vi "Autonomous Independent.vi"() -> ()   [LabVIEW 2019]
doc: "This VI is called when autonomous begins, and will automatically be terminated when autonomous ends. You can carry out timed or sensor driven robot movement independently without needing to return to the caller."
uses:
  <vilib>/Rock Robotics/WPI/Utilities/WPI_GetSetVariantRefNum.vi
  <vilib>/Rock Robotics/Network Tables/NT Read String.vi
  <vilib>/Rock Robotics/Network Tables/NT Write Numeric Array.vi
  Robot Global Data.vi
  <vilib>/Rock Robotics/WPI/RobotDrive/WPI_RobotDriveArcadeDrive_Standard(NoSaturation).vi
panel:
  out "time":u32
  # "Be sure to right-click and choose Data Operations>>Make Current Value default if you want to save the array values with the VI"
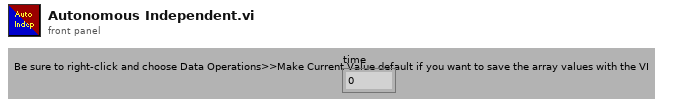
[diagram p1: front panel]
types:
  T1 = typedef "WPI_JoystickDevRef.ctl" = cluster{"Device":T2}
  T2 = typedef "WPI_JoystickDeviceEnum.ctl" = enum16{"USB 0", "USB 1", "USB 2", "USB 3", "USB 4", "USB 5"}
  T3 = typedef "WPI_MotorControlDeviceRef.ctl" = cluster{"DeviceStatus":errorcluster, "Type":T4, "PWM":cluster{"PWM Channel":T5, "DeadBand":T6}, "CAN":cluster{"Device Number":u8, "SetOutput VI Ref":variant, "GetOutput VI Ref":variant, "Enable VI Ref":variant, "Disable VI Ref":variant, "Data":variant}, "Invert":bool, "DIO PWM":cluster{"PWM \"Enable\" Channel":T5, "DIOChannel":T7, "PWM Rate":dbl}}
  T4 = typedef "WPI_MotorControlType.ctl" = enum16{"PWM", "CAN", "DIO PWM"}
  T5 = typedef "FPGA_DIOPWMChannel.ctl" = enum8{"PWM 0", "PWM 1", "PWM 2", "PWM 3", "PWM 4", "PWM 5", "PWM 6", "PWM 7", "PWM 8", "PWM 9", "PWM MXP 0", "PWM MXP 1", "PWM MXP 2", "PWM MXP 3", "PWM MXP 4", "PWM MXP 5", "PWM MXP 6", "PWM MXP 7", "PWM MXP 8", "PWM MXP 9", "Invalid"}
  T6 = typedef "WPI_PWMDeadband.ctl" = cluster{"Name":string, "maxPositivePwm":i32, "minPositivePwm":i32, "centerPwm":i32, "maxNegativePwm":i32, "minNegativePwm":i32, "angularRange":u16}
  T7 = typedef "FPGA_DIOChannel.ctl" = enum8{"DIO 0", "DIO 1", "DIO 2", "DIO 3", "DIO 4", "DIO 5", "DIO 6", "DIO 7", "DIO 8", "DIO 9", "DIO MXP 0", "DIO MXP 1", "DIO MXP 2", "DIO MXP 3", "DIO MXP 4", "DIO MXP 5", "DIO MXP 6", "DIO MXP 7", "DIO MXP 8", "DIO MXP 9", "DIO MXP 10", "DIO MXP 11", "DIO MXP 12", "DIO MXP 13", "DIO MXP 14", "DIO MXP 15", "SPI Port CS1", "SPI Port CS2", "SPI Port CS3", "SPI Port MISO", "SPI Port MOSI", "Invalid"}
  T8 = typedef "WPI_RobotDriveDevRef.ctl" = cluster{"DevStatus":errorcluster, "Motors[]":T3[], "Square Inputs":bool, "Max Output":dbl}
  T9 = cluster{"offsetAngle H":dbl, "offsetAngle V":dbl, "area":dbl, "skew":dbl, "target":dbl}
  T10 = cluster{"Yaw":dbl, "Roll":dbl, "Pitch":dbl, "Heading":dbl, "Fused Heading":dbl}
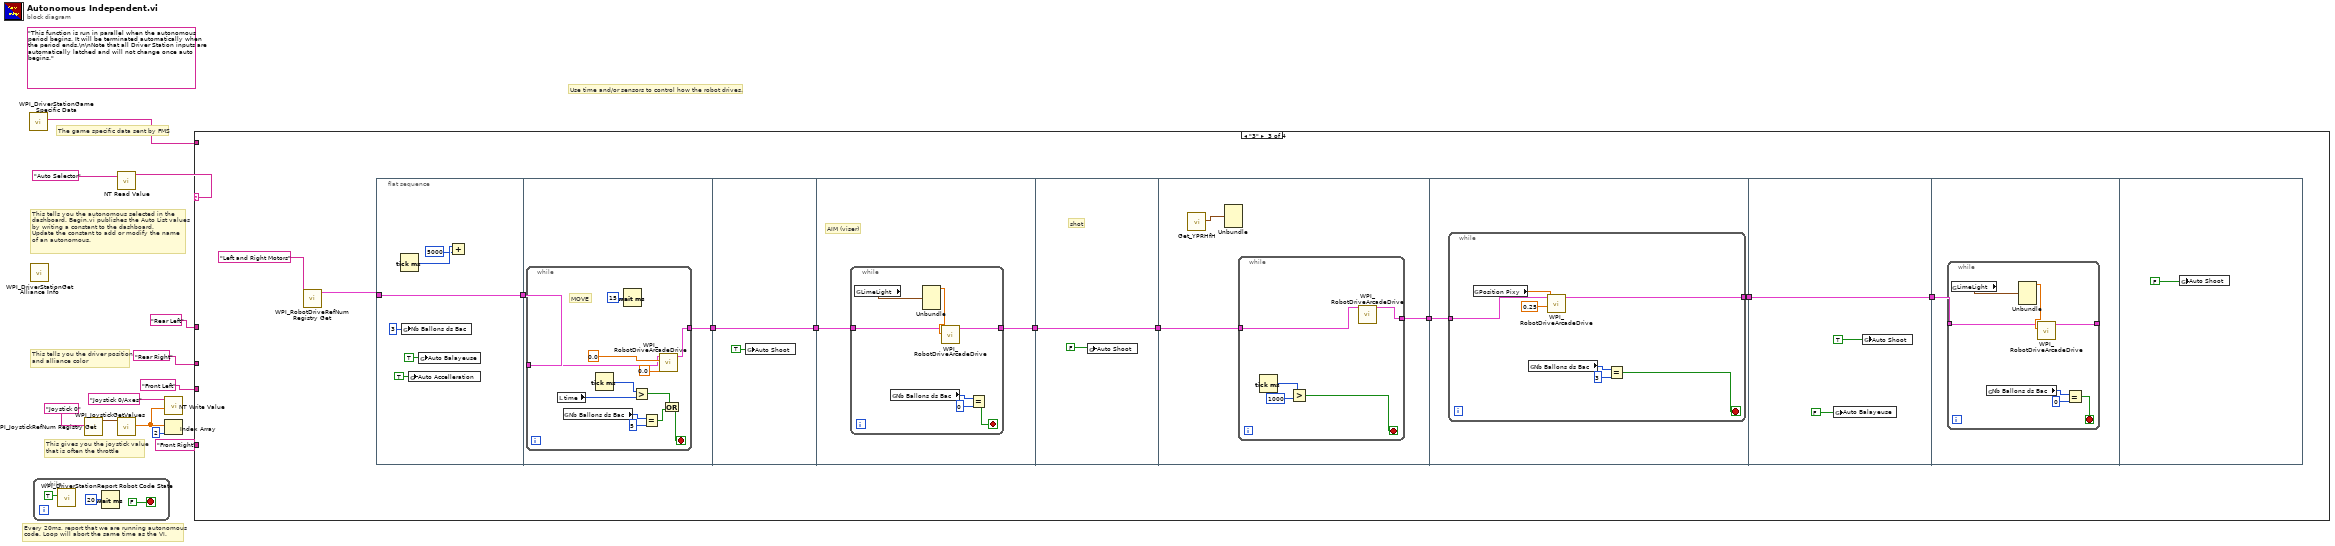
[diagram p0: block diagram]
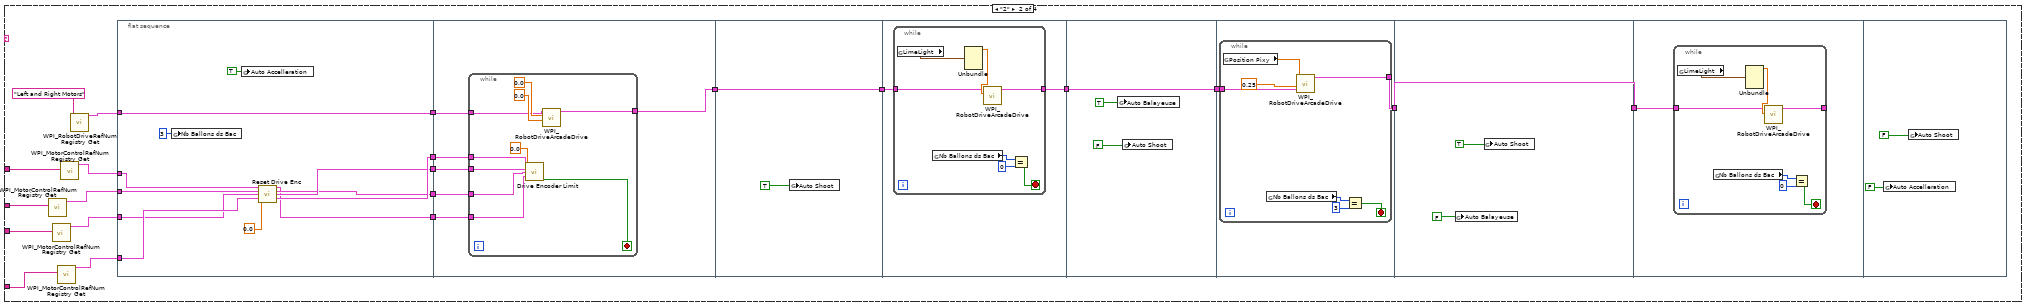
[diagram p3: hidden frame]
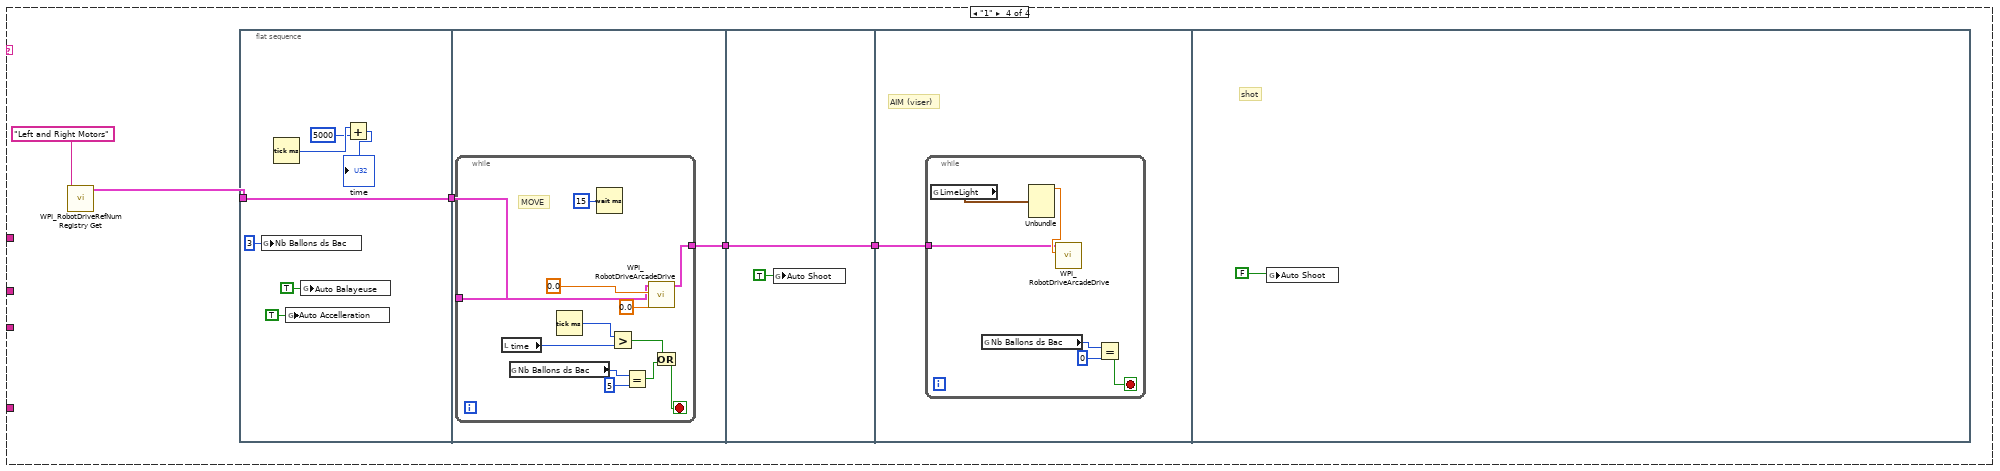
[diagram p4: hidden frame]
diagram:
  (unwired) "This function is run in parallel when the autonomous period begins. It will be terminated automatically when the period ends.\n\nNote that all Driver Station inputs are automatically latched and will not change once auto begins."
  # "The game specific data sent by FMS"
  # "This tells you the autonomous selected in the \ndashboard. Begin.vi publishes the Auto List values\nby writing a constant to the dashboard.\nUpdate the constant to add or modify the name\nof an autonomous."
  # "Every 20ms, report that we are running autonomous\ncode. Loop will abort the same time as the VI."
  # "This gives you the joystick value\nthat is often the throttle"
  # "Use time and/or sensors to control how the robot drives."
  # "This tells you the driver position\nand alliance color"
  n1 = call <vilib>:"WPI_DriverStationGame Specific Data.vi"() -> ("Game Specific Data"=w5:string)  [unwired: 11 in]
  n2 = call <vilib>:"WPI_DriverStationGet Alliance Info.vi"() -> ()  [unwired: 12 out]
  n3 = while {
    stop <- FALSE stop-if-true
    n4 = call <vilib>:"WPI_DriverStationReport Robot Code State.vi"("Autonomous"=TRUE) -> ()  [unwired: 10 in, 1 out]
    n5 = Wait (ms)(milliseconds to wait=u32 20) -> ()  [unwired: 1 out]
  }
  n6 = call <vilib>:"WPI_JoystickRefNum Registry Get.vi"("refnum name"="Joystick 0") -> ("JoystickDevRef"=w11:T1)  [unwired: 1 in, 9 out]
  n7 = call <vilib>:"WPI_JoystickGetValues.vi"("JoystickDevRef"=w11) -> ("Axes"=w7:dbl[])  [unwired: 6 in, 4 out]
  n8 = call-poly <vilib>:"NT Read Value.vi"("Name"="Auto Selector") -> ("String"=w8:string)  [unwired: 9 in, 1 out]
  n9 = call-poly <vilib>:"NT Write Value.vi"("Numeric Array"=w7, "Name"="Joystick 0/Axes") -> ()  [unwired: 9 in, 1 out]
  n10 = Index Array(array=w7, index=2) -> ()  [unwired: 1 out]
  n11 = case shown="\"3\"" w8 {
    tunnel: w5 -> [_ _ _ _]
    tunnel: "Rear Left" ("refnum name") -> [_ w20 _ _]
    tunnel: "Rear Right" ("refnum name") -> [_ w19 _ _]
    tunnel: "Front Left" ("refnum name") -> [_ w18 _ _]
    tunnel: "Front Right" ("refnum name") -> [_ w17 _ _]
    frame Default {
      # "You can put your main auto here, or you can right-click on the case and make any\nother frame be the default case."
      # "This is the frame that will execute if no selection is made, or if it is not recognized"
    }
    frame "2" {
      n12 = call <vilib>:"WPI_MotorControlRefNum Registry Get.vi"("refnum name"=w19) -> ("MotorControlDevRef"=w34:T3)  [unwired: 9 in, 1 out]
      n13 = call <vilib>:"WPI_MotorControlRefNum Registry Get.vi"("refnum name"=w18) -> ("MotorControlDevRef"=w33:T3)  [unwired: 9 in, 1 out]
      n14 = call <vilib>:"WPI_MotorControlRefNum Registry Get.vi"("refnum name"=w17) -> ("MotorControlDevRef"=w32:T3)  [unwired: 9 in, 1 out]
      n15 = call <vilib>:"WPI_MotorControlRefNum Registry Get.vi"("refnum name"=w20) -> ("MotorControlDevRef"=w35:T3)  [unwired: 9 in, 1 out]
      n16 = call <vilib>:"WPI_RobotDriveRefNum Registry Get.vi"("refnum name"="Left and Right Motors") -> ("RobotDriveDevRef"=w36:T8)  [unwired: 9 in, 1 out]
      n17 = flat-sequence {
        tunnel: w36 -> [w48]
        tunnel: w35 -> [w40]
        tunnel: w34 -> [w41]
        tunnel: w33 -> [w42]
        tunnel: w32 -> [w47]
        tunnel: [w44] -> w31
        tunnel: [w43] -> w30
        tunnel: [w48] -> w29
        tunnel: [w46] -> w28
        tunnel: [w45] -> w27
        tunnel: w31 -> [w52]
        tunnel: w30 -> [w51]
        tunnel: w29 -> [w50]
        tunnel: w28 -> [w54]
        tunnel: w27 -> [w53]
        tunnel: [w49] -> w26
        tunnel: w26 -> [w66]
        tunnel: [w66] -> w25
        tunnel: w25 -> [w68]
        tunnel: [w67] -> w23
        tunnel: [w76] -> w24
        tunnel: w23 -> [w76]
        tunnel: w24 -> [w80]
        tunnel: [w79] -> w22
        tunnel: w22 -> [w89]
        tunnel: [w89] -> w21
        tunnel: w21 -> [w91]
        frame #0 {
          n18 = global write "Robot Global Data.vi" "Nb Ballons ds Bac"(u8 3 ("Nb Ballons ds Bac")) -> ()
          n19 = global write "Robot Global Data.vi" "Auto Accelleration"(TRUE ("Auto Accelleration")) -> ()
          n20 = call "Reset Drive Enc.vi"("MotorControlDevRef"=w40, "MotorControlDevRef 2"=w41, "MotorControlDevRef 3"=w42, "MotorControlDevRef 4"=w47, "Position"=0.0) -> ("MotorControlDeviceRef"=w43:T3, "MotorControlDeviceRef 2"=w44:T3, "MotorControlDeviceRef 3"=w45:T3, "MotorControlDeviceRef 4"=w46:T3)  [unwired: 7 in]
        }
        frame #1 {
          n21 = while {
            tunnel: w54 -> [w64]
            tunnel: w53 -> [w63]
            tunnel: w52 -> [w62]
            tunnel: w51 -> [w61]
            tunnel: w50 -> [w56]
            tunnel: [w55] -> w49
            stop <- w60 stop-if-true
            n22 = call "Drive Encoder Limit.vi"("MotorControlDevRef"=w64, "MotorControlDevRef 2"=w63, "MotorControlDevRef 3"=w62, "MotorControlDevRef 4"=w61, "Limit"=0.0) -> ("Limit Triggered"=w60:bool)  [unwired: 6 in, 4 out]
            n23 = call-poly <vilib>:"WPI_RobotDriveArcadeDrive.vi"("Y axis value"=0.0, "X axis value"=0.0, "RobotDriveDevRef"=w56) -> ("RobotDriveDevRef"=w55:T8)  [unwired: 6 in, 2 out]
          }
        }
        frame #2 {
          n24 = global write "Robot Global Data.vi" "Auto Shoot"(TRUE ("Auto Balayeuse")) -> ()
        }
        frame #3 {
          n25 = while {
            tunnel: w68 -> [w70]
            tunnel: [w69] -> w67
            stop <- w73 stop-if-true
            n26 = global read "Robot Global Data.vi" "LimeLight"() -> (w72:T9)
            n27 = global read "Robot Global Data.vi" "Nb Ballons ds Bac"() -> (w75:u8)
            n28 = Unbundle(w72) -> ("offsetAngle H"=w71:dbl)  [unwired: 4 out]
            n29 = call-poly <vilib>:"WPI_RobotDriveArcadeDrive.vi"("X axis value"=w71, "RobotDriveDevRef"=w70) -> ("RobotDriveDevRef"=w69:T8)  [unwired: 7 in, 2 out]
            n30 = Equal?(x=w75, y=u8 0) -> (x = y?=w73:bool)
          }
        }
        frame #4 {
          n31 = global write "Robot Global Data.vi" "Auto Balayeuse"(TRUE ("Auto Balayeuse")) -> ()
          n32 = global write "Robot Global Data.vi" "Auto Shoot"(FALSE ("Auto Balayeuse")) -> ()
        }
        frame #5 {
          n33 = while {
            tunnel: [w87] -> w79
            tunnel: w80 -> [w86]
            stop <- w81 stop-if-true
            n34 = global read "Robot Global Data.vi" "Position Pixy"() -> (w85:dbl)
            n35 = global read "Robot Global Data.vi" "Nb Ballons ds Bac"() -> (w83:u8)
            n36 = call-poly <vilib>:"WPI_RobotDriveArcadeDrive.vi"("Y axis value"=0.25, "X axis value"=w85, "RobotDriveDevRef"=w86) -> ("RobotDriveDevRef"=w87:T8)  [unwired: 6 in, 2 out]
            n37 = Equal?(x=w83, y=u8 3) -> (x = y?=w81:bool)
          }
        }
        frame #6 {
          n38 = global write "Robot Global Data.vi" "Auto Balayeuse"(FALSE ("Auto Balayeuse")) -> ()
          n39 = global write "Robot Global Data.vi" "Auto Shoot"(TRUE ("Auto Balayeuse")) -> ()
        }
        frame #7 {
          n40 = while {
            tunnel: w91 -> [w93]
            tunnel: [w92] -> _
            stop <- w96 stop-if-true
            n41 = global read "Robot Global Data.vi" "LimeLight"() -> (w95:T9)
            n42 = global read "Robot Global Data.vi" "Nb Ballons ds Bac"() -> (w98:u8)
            n43 = Unbundle(w95) -> ("offsetAngle H"=w94:dbl)  [unwired: 4 out]
            n44 = call-poly <vilib>:"WPI_RobotDriveArcadeDrive.vi"("X axis value"=w94, "RobotDriveDevRef"=w93) -> ("RobotDriveDevRef"=w92:T8)  [unwired: 7 in, 2 out]
            n45 = Equal?(x=w98, y=u8 0) -> (x = y?=w96:bool)
          }
        }
        frame #8 {
          n46 = global write "Robot Global Data.vi" "Auto Accelleration"(FALSE ("Auto Balayeuse")) -> ()
          n47 = global write "Robot Global Data.vi" "Auto Shoot"(FALSE ("Auto Balayeuse")) -> ()
        }
      }
    }
    frame "3" {
      n48 = call <vilib>:"WPI_RobotDriveRefNum Registry Get.vi"("refnum name"="Left and Right Motors") -> ("RobotDriveDevRef"=w107:T8)  [unwired: 9 in, 1 out]
      n49 = flat-sequence {
        tunnel: [w116] -> w110
        tunnel: w107 -> [w116]
        tunnel: w110 -> [w118]
        tunnel: [w117] -> w109
        tunnel: w109 -> [w131]
        tunnel: [w131] -> w108
        tunnel: w108 -> [w134]
        tunnel: [w133] -> w105
        tunnel: [w142] -> w106
        tunnel: w105 -> [w142]
        tunnel: w106 -> [w146]
        tunnel: [w144] -> w103
        tunnel: w103 -> [w153]
        tunnel: [w152] -> w101
        tunnel: [w161] -> w102
        tunnel: w101 -> [w161]
        tunnel: w102 -> [w164]
        frame #0 {
          n50 = Tick Count (ms)() -> (millisecond timer value=w113:u32)
          n51 = global write "Robot Global Data.vi" "Nb Ballons ds Bac"(u8 3 ("Nb Ballons ds Bac")) -> ()
          n52 = global write "Robot Global Data.vi" "Auto Accelleration"(TRUE ("Auto Accelleration")) -> ()
          n53 = global write "Robot Global Data.vi" "Auto Balayeuse"(TRUE ("Auto Balayeuse")) -> ()
          n54 = Add(x=w113, y=u32 5000) -> ()  [unwired: 1 out]
        }
        frame #1 {
          n55 = while {
            tunnel: w118 -> [w128]
            tunnel: [w119] -> w117
            stop <- w120 stop-if-true
            # "MOVE"
            n56 = local read "time"() -> (w123:u32)
            n57 = global read "Robot Global Data.vi" "Nb Ballons ds Bac"() -> (w127:u8)
            n58 = Tick Count (ms)() -> (millisecond timer value=w124:u32)
            n59 = Wait (ms)(milliseconds to wait=u32 15) -> ()  [unwired: 1 out]
            n60 = Greater?(x=w124, y=w123) -> (0:w121:bool)
            n61 = Equal?(x=w127, y=u8 5) -> (x = y?=w122:bool)
            n62 = call-poly <vilib>:"WPI_RobotDriveArcadeDrive.vi"("Y axis value"=0.0, "X axis value"=0.0, "RobotDriveDevRef"=w128) -> ("RobotDriveDevRef"=w119:T8)  [unwired: 6 in, 2 out]
            n63 = Or(x=w121, y=w122) -> (x .or. y?=w120:bool)
          }
        }
        frame #2 {
          n64 = global write "Robot Global Data.vi" "Auto Shoot"(TRUE ("Auto Shoot")) -> ()
        }
        frame #3 {
          # "AIM (viser)"
          n65 = while {
            tunnel: w134 -> [w136]
            tunnel: [w135] -> w133
            stop <- w139 stop-if-true
            n66 = global read "Robot Global Data.vi" "LimeLight"() -> (w138:T9)
            n67 = global read "Robot Global Data.vi" "Nb Ballons ds Bac"() -> (w141:u8)
            n68 = Unbundle(w138) -> ("offsetAngle H"=w137:dbl)  [unwired: 4 out]
            n69 = call-poly <vilib>:"WPI_RobotDriveArcadeDrive.vi"("X axis value"=w137, "RobotDriveDevRef"=w136) -> ("RobotDriveDevRef"=w135:T8)  [unwired: 7 in, 2 out]
            n70 = Equal?(x=w141, y=u8 0) -> (x = y?=w139:bool)
          }
        }
        frame #4 {
          # "shot"
          n71 = global write "Robot Global Data.vi" "Auto Shoot"(FALSE) -> ()
        }
        frame #5 {
          n72 = call <vilib>:"Get_YPRHfH.vi"() -> ("YRPHfH"=w145:T10)  [unwired: 11 in]
          n73 = Unbundle(w145) -> ()  [unwired: 5 out]
          n74 = while {
            tunnel: w146 -> [w151]
            tunnel: [w150] -> w144
            stop <- w147 stop-if-true
            n75 = Tick Count (ms)() -> (millisecond timer value=w149:u32)
            n76 = Greater?(x=w149, y=u32 1000) -> (0:w147:bool)
            n77 = call-poly <vilib>:"WPI_RobotDriveArcadeDrive.vi"("RobotDriveDevRef"=w151) -> ("RobotDriveDevRef"=w150:T8)  [unwired: 8 in, 2 out]
          }
        }
        frame #6 {
          n78 = while {
            tunnel: w153 -> [w160]
            tunnel: [w154] -> w152
            stop <- w155 stop-if-true
            n79 = global read "Robot Global Data.vi" "Position Pixy"() -> (w159:dbl)
            n80 = global read "Robot Global Data.vi" "Nb Ballons ds Bac"() -> (w157:u8)
            n81 = call-poly <vilib>:"WPI_RobotDriveArcadeDrive.vi"("Y axis value"=0.25, "X axis value"=w159, "RobotDriveDevRef"=w160) -> ("RobotDriveDevRef"=w154:T8)  [unwired: 6 in, 2 out]
            n82 = Equal?(x=w157, y=u8 3) -> (x = y?=w155:bool)
          }
        }
        frame #7 {
          n83 = global write "Robot Global Data.vi" "Auto Balayeuse"(FALSE ("Auto Balayeuse")) -> ()
          n84 = global write "Robot Global Data.vi" "Auto Shoot"(TRUE ("Auto Balayeuse")) -> ()
        }
        frame #8 {
          n85 = while {
            tunnel: w164 -> [w167]
            tunnel: [w166] -> _
            stop <- w165 stop-if-true
            n86 = global read "Robot Global Data.vi" "LimeLight"() -> (w169:T9)
            n87 = global read "Robot Global Data.vi" "Nb Ballons ds Bac"() -> (w171:u8)
            n88 = Unbundle(w169) -> ("offsetAngle H"=w168:dbl)  [unwired: 4 out]
            n89 = call-poly <vilib>:"WPI_RobotDriveArcadeDrive.vi"("X axis value"=w168, "RobotDriveDevRef"=w167) -> ("RobotDriveDevRef"=w166:T8)  [unwired: 7 in, 2 out]
            n90 = Equal?(x=w171, y=u8 0) -> (x = y?=w165:bool)
          }
        }
        frame #9 {
          n91 = global write "Robot Global Data.vi" "Auto Shoot"(FALSE ("Auto Balayeuse")) -> ()
        }
      }
    }
    frame "1" {
      n92 = call <vilib>:"WPI_RobotDriveRefNum Registry Get.vi"("refnum name"="Left and Right Motors") -> ("RobotDriveDevRef"=w176:T8)  [unwired: 9 in, 1 out]
      n93 = flat-sequence {
        tunnel: [w184] -> w177
        tunnel: w176 -> [w184]
        tunnel: w177 -> [w186]
        tunnel: [w185] -> w175
        tunnel: w175 -> [w199]
        tunnel: [w199] -> w174
        tunnel: w174 -> [w201]
        frame #0 {
          n94 = global write "Robot Global Data.vi" "Nb Ballons ds Bac"(u8 3 ("Nb Ballons ds Bac")) -> ()
          n95 = Tick Count (ms)() -> (millisecond timer value=w181:u32)
          n96 = global write "Robot Global Data.vi" "Auto Accelleration"(TRUE ("Auto Accelleration")) -> ()
          n97 = global write "Robot Global Data.vi" "Auto Balayeuse"(TRUE ("Auto Balayeuse")) -> ()
          n98 = Add(x=w181, y=u32 5000) -> (x+y=→"time":u32)
        }
        frame #1 {
          n99 = while {
            tunnel: w186 -> [w196]
            tunnel: [w187] -> w185
            stop <- w188 stop-if-true
            # "MOVE"
            n100 = local read "time"() -> (w191:u32)
            n101 = global read "Robot Global Data.vi" "Nb Ballons ds Bac"() -> (w195:u8)
            n102 = Tick Count (ms)() -> (millisecond timer value=w192:u32)
            n103 = Wait (ms)(milliseconds to wait=u32 15) -> ()  [unwired: 1 out]
            n104 = Greater?(x=w192, y=w191) -> (0:w189:bool)
            n105 = Equal?(x=w195, y=u8 5) -> (x = y?=w190:bool)
            n106 = call-poly <vilib>:"WPI_RobotDriveArcadeDrive.vi"("Y axis value"=0.0, "X axis value"=0.0, "RobotDriveDevRef"=w196) -> ("RobotDriveDevRef"=w187:T8)  [unwired: 6 in, 2 out]
            n107 = Or(x=w189, y=w190) -> (x .or. y?=w188:bool)
          }
        }
        frame #2 {
          n108 = global write "Robot Global Data.vi" "Auto Shoot"(TRUE ("Auto Shoot")) -> ()
        }
        frame #3 {
          # "AIM (viser)"
          n109 = while {
            tunnel: w201 -> [w202]
            stop <- w205 stop-if-true
            n110 = global read "Robot Global Data.vi" "LimeLight"() -> (w204:T9)
            n111 = global read "Robot Global Data.vi" "Nb Ballons ds Bac"() -> (w207:u8)
            n112 = Unbundle(w204) -> ("offsetAngle H"=w203:dbl)  [unwired: 4 out]
            n113 = call-poly <vilib>:"WPI_RobotDriveArcadeDrive.vi"("X axis value"=w203, "RobotDriveDevRef"=w202) -> ()  [unwired: 7 in, 3 out]
            n114 = Equal?(x=w207, y=u8 0) -> (x = y?=w205:bool)
          }
        }
        frame #4 {
          # "shot"
          n115 = global write "Robot Global Data.vi" "Auto Shoot"(FALSE) -> ()
        }
      }
    }
  }
